vi "Package ID to JSON.vi"(11 "Package":T1) -> (3 "Package JSON":string)   [LabVIEW 2020, in "neg-pkg.lvlib" / "Package.lvclass"]
uses:
  Package.lvclass
  Package ID.ctl
  Package Type.ctl
  neg_pkgs/negentropicdev/lv-json/JSON/JSON.lvlib
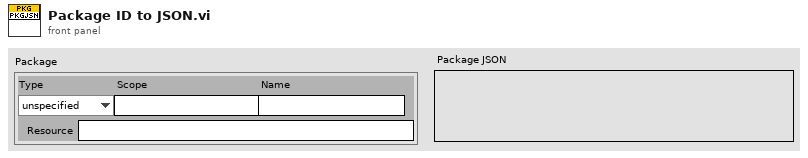
[diagram p1: front panel]
types:
  T1 = typedef "neg-pkg.lvlib/Package.lvclass/Package ID.ctl" = cluster{"Type":T2, "Scope":string, "Name":string, "Resource":string}
  T2 = typedef "neg-pkg.lvlib/Package.lvclass/Package Type.ctl" = enum16{"unspecified", "git"}
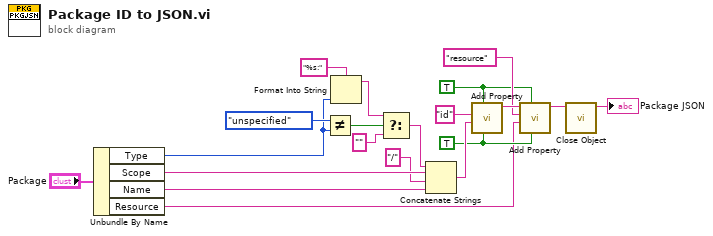
[diagram p0: block diagram]
diagram:
  w4 = TRUE ("String?")
  w5 = TRUE ("Include Empty?")
  n1 = Unbundle By Name("Package") -> ("Type"=w18:T2, "Scope"=w12:string, "Name"=w13:string, "Resource"=w3:string)
  n2 = Not Equal?(x=Package_Type."unspecified", y=w18) -> (x != y?=w17:bool)
  n3 = Format Into String(format string="%s:", w18) -> (resulting string=w15:string)  [unwired: 2 in, 1 out]
  n4 = Select(t=w15, s=w17, f="") -> (s? t:f=w11:string)
  n5 = Concatenate Strings(w11, w12, "/" ("string"), w13) -> (w9:string)
  n6 = call "Add Property.vi"("String?"=w4, "Include Empty?"=w5, "Value"=w9, "Property Name"="id") -> ("String out"=w7:string)  [unwired: 7 in]
  n7 = call "Add Property.vi"("String?"=w4, "Include Empty?"=w5, "Value"=w3, "Property Name"="resource", "String In"=w7) -> ("String out"=w2:string)  [unwired: 6 in]
  n8 = call "Close Object.vi"("String In"=w2) -> ("String out"=→"Package JSON":string)  [unwired: 10 in]
